vi "Read SRFF Spectrum.vi"(8 "error in (no error)":errorcluster, 11 "Analyze Results FF-Spectrum in":refnum<class "Analyze Results FF-Spectrum.lvclass">) -> (0 "error out":errorcluster, 2 "SRFF Spectrum":T1[](array[typedef]), 3 "Analyze Results FF-Spectrum out":refnum<class "Analyze Results FF-Spectrum.lvclass">)   [LabVIEW 2014, in "Analyze Results FF-Spectrum.lvclass"]
uses:
  Analyze Results FF-Spectrum.lvclass
  Spectral Point.ctl
  Analyze Results FF-Spectrum.lvclass/Analyze Results FF-Spectrum.ctl
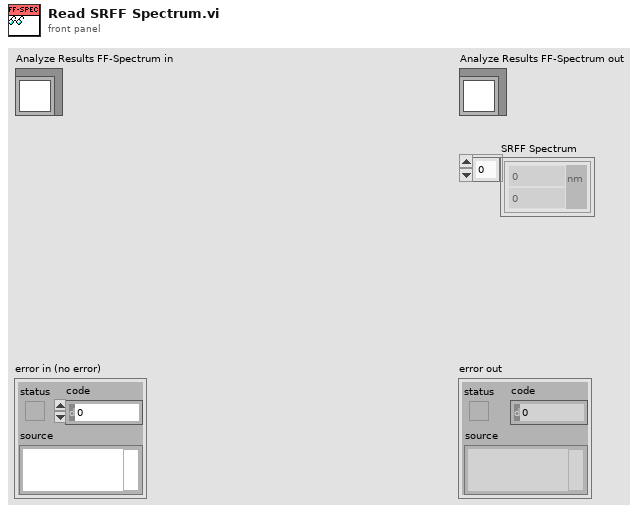
[diagram p1: front panel]
types:
  T1 = typedef "Analyze Results FF-Spectrum.lvclass/Spectral Point.ctl" = cluster{dbl[unit], dbl}
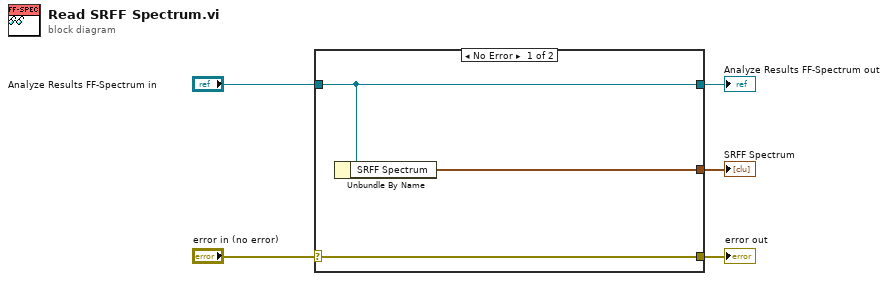
[diagram p0: block diagram]
diagram:
  n1 = case shown="No Error" "error in (no error)" {
    selector: "error in (no error)" -> [w8 w9]
    tunnel: [w8 w9] -> w4
    tunnel: [w7 w10] -> w2
    tunnel: "Analyze Results FF-Spectrum in" -> [w7 w10]
    tunnel: [w6 _] -> w1
    frame No Error {
      n2 = Unbundle By Name(w7) -> ("SRFF Spectrum"=w6:T1[])
    }
    frame Error {
    }
  }
  "error out" <- w4
  "Analyze Results FF-Spectrum out" <- w2
  "SRFF Spectrum" <- w1
